vi "CalcDivergence.vi"(6 "AOI":cluster{"AOI h, px":dbl, "AOI w, px":dbl}, 7 "Rotate, deg":dbl=1.6 format="%#_13g", 8 "Focus, mm":dbl=192.0, 9 "Pixel size, um":dbl=6.45, 10 "Threshold, %":dbl=85.0 format="%#_13g", 11 "path to file":path=path "E:/New folder (3)/Laser(3dots)_FarField_after_Passive(WO_SAC).png") -> (2 "Slow Axis":T1, 3 "Fast Axis":T1)   [LabVIEW 2017]
panel:
  out "Picture":picture
  in  "Zoom Factor":sgl=0.4
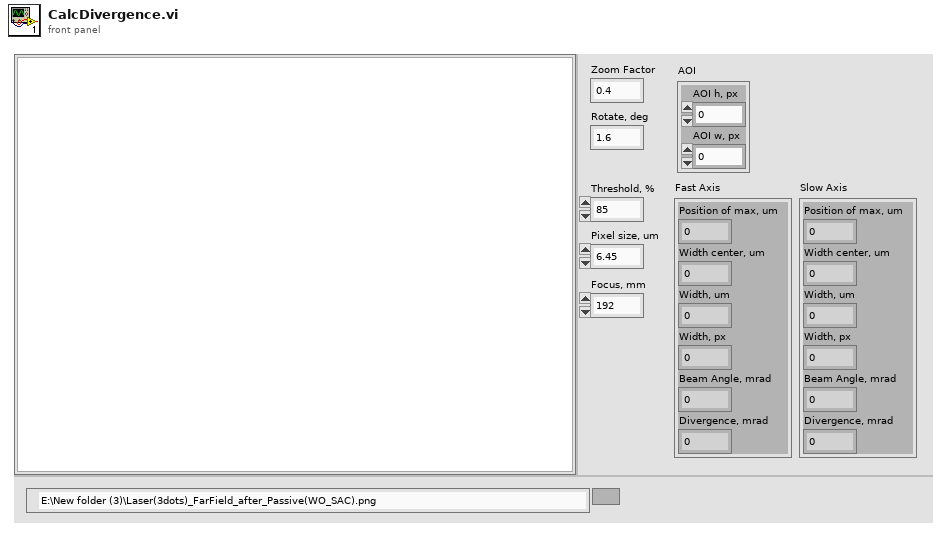
[diagram p1: front panel]
types:
  T1 = cluster{"Position of max, um":dbl, "Width center, um":dbl, "Width, um":dbl, "Width, px":i32, "Beam Angle, mrad":dbl, "Divergence, mrad":dbl}
  T2 = typedef "imagedata.ctl" = cluster{"image type":i32, "image depth":i32, "image":u8[], "mask":u8[], "colors":u32[], "Rectangle":cluster{"left":i16, "top":i16, "right":i16, "bottom":i16}}
  T3 = cluster{"Centroid of max, um":dbl, "Centroid of width, um":dbl, "Width, um":dbl, "Width, px":i32, "Beam Angle, mrad":dbl, "Divergence, mrad":dbl}
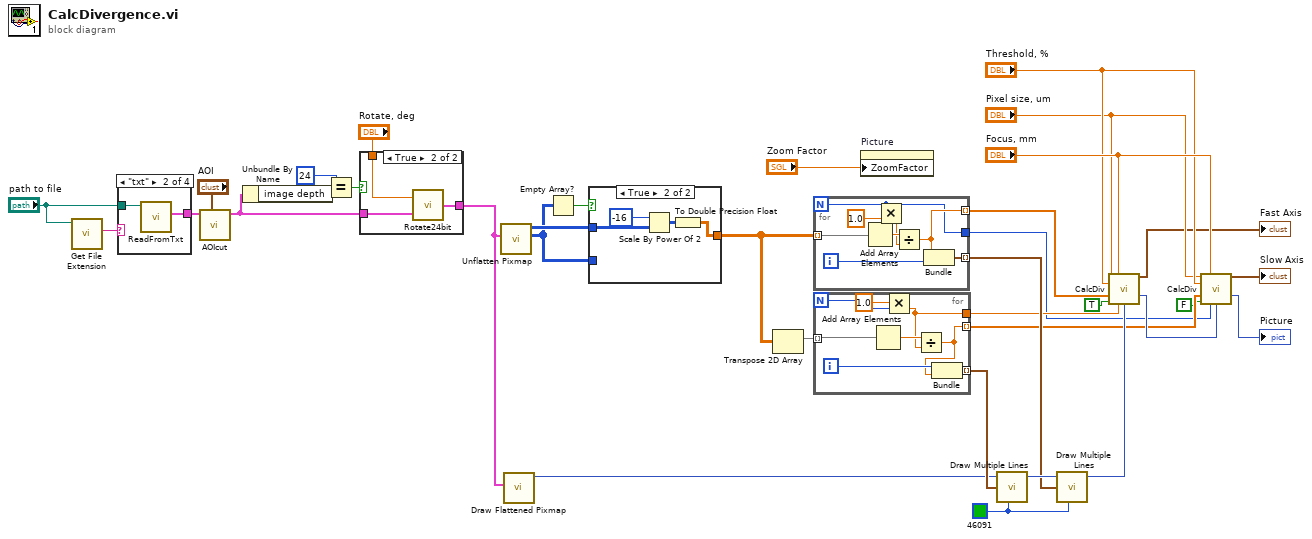
[diagram p0: block diagram]
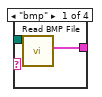
[diagram p2: hidden frame]
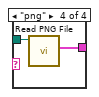
[diagram p4: hidden frame]
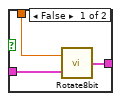
[diagram p5: hidden frame]
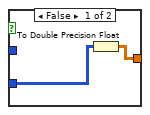
[diagram p6: hidden frame]
diagram:
  w26 = u32 46091 ("color(black)")
  n1 = call <vilib>:"Get File Extension.vi"("file"="path to file") -> ("lowercase file extension"=w7:string)  [unwired: 6 in, 4 out]
  n2 = case shown="\"txt\"" w7 {
    tunnel: [w36 w38 _ w41] -> w6
    tunnel: "path to file" -> [w37 w39 _ w40]
    frame "bmp" {
      n3 = call <vilib>:"Read BMP File.vi"("path to BMP file"=w37) -> ("image data"=w36:T2)  [unwired: 8 in, 2 out]
    }
    frame "txt" {
      n4 = call "ReadFromTxt.vi"("path to PNG file"=w39) -> ("image data"=w38:T2)  [unwired: 10 in]
    }
    frame Default {
    }
    frame "png" {
      n5 = call <vilib>:"Read PNG File.vi"("path to PNG file"=w40) -> ("image data"=w41:T2)  [unwired: 8 in, 2 out]
    }
  }
  n6 = call "AOIcut.vi"("AOI"="AOI", "image data in"=w6) -> ("image data out"=w3:T2)  [unwired: 9 in]
  n7 = Unbundle By Name(w3) -> ("image depth"=w10:i32)
  n8 = Equal?(x=24, y=w10) -> (x = y?=w8:bool)
  n9 = case shown="True" w8 {
    tunnel: "Rotate, deg" -> [w44 w47]
    tunnel: [w42 w46] -> w30
    tunnel: w3 -> [w43 w45]
    frame False {
      n10 = call "Rotate8bit.vi"("image data"=w43, "theta (deg)"=w44) -> ("image data 2"=w42:T2)
    }
    frame True {
      n11 = call "Rotate24bit.vi"("image data"=w45, "theta (deg)"=w47) -> ("image data 2"=w46:T2)
    }
  }
  n12 = call <vilib>:"Unflatten Pixmap.vi"("image data"=w30) -> ("8-bit pixmap"=w12:u8[][], "24-bit pixmap"=w14:u32[][])  [unwired: 4 in, 5 out]
  n13 = call <vilib>:"Draw Flattened Pixmap.vi"("image data"=w30) -> ("new picture"=w29:picture)  [unwired: 8 in]
  n14 = Empty Array?(array=w12) -> (empty?=w11:bool)
  n15 = case shown="True" w11 {
    tunnel: w14 -> [_ w53]
    tunnel: [w49 w50] -> w13
    tunnel: w12 -> [w48 _]
    frame False {
      n16 = To Double Precision Float(number=w48) -> (double precision float=w49:dbl[][])
    }
    frame True {
      n17 = Scale By Power Of 2(n=i16 -16, x=w53) -> (x*2^n=w51:u32[][])
      n18 = To Double Precision Float(number=w51) -> (double precision float=w50:dbl[][])
    }
  }
  n19 = Transpose 2D Array(2D array=w13) -> (transposed array=w33:dbl[][])
  n20 = for {
    N -> [w57]
    tunnel: w13 -> [w56] mode=indexing
    tunnel: [w60] -> w28 mode=indexing
    tunnel: [w58] -> w25 mode=indexing
    tunnel: [w57] -> w19
    i -> [w61]
    n21 = Add Array Elements(numeric array=w56) -> (sum=w59:dbl)
    n22 = Multiply(x=w57, y=1.0) -> (x*y=w55:dbl)
    n23 = Divide(x=w59, y=w55) -> (x/y=w58:dbl)
    n24 = Bundle(w58, w61) -> (w60:cluster{dbl, i32})  [unwired: 1 in]
  }
  n25 = for {
    N -> [w66]
    tunnel: w33 -> [w64] mode=indexing
    tunnel: [w68] -> w32 mode=indexing
    tunnel: [w63] -> w24
    tunnel: [w65] -> w20 mode=indexing
    i -> [w69]
    n26 = Add Array Elements(numeric array=w64) -> (sum=w67:dbl)
    n27 = Multiply(x=1.0, y=w66) -> (x*y=w63:dbl)
    n28 = Divide(x=w67, y=w63) -> (x/y=w65:dbl)
    n29 = Bundle(w69, w65) -> (w68:cluster{i32, dbl})  [unwired: 1 in]
  }
  n30 = property on="Picture" class="Pict"("ZoomFactor"="Zoom Factor") -> ()  [unwired: 2 in, 2 out]
  n31 = call <vilib>:"Draw Multiple Lines.vi"("picture"=w29, "line endpoints"=w32, "color(black)"=w26) -> ("new picture"=w31:picture)  [unwired: 6 in]
  n32 = call <vilib>:"Draw Multiple Lines.vi"("picture"=w31, "line endpoints"=w28, "color(black)"=w26) -> ("new picture"=w27:picture)  [unwired: 6 in]
  n33 = call "CalcDiv.vi"("Pixel size, um"="Pixel size, um", "Focus, mm"="Focus, mm", "Threshold, %"="Threshold, %", "Array"=w25, "SAC/FAC"=TRUE, "Numeric in"=w24, "new picture in"=w27) -> ("Beam Params"=→"Fast Axis":T3, "new picture out"=w23:picture)  [unwired: 7 in]
  n34 = call "CalcDiv.vi"("Pixel size, um"="Pixel size, um", "Focus, mm"="Focus, mm", "Threshold, %"="Threshold, %", "Array"=w20, "SAC/FAC"=FALSE, "Numeric in"=w19, "new picture in"=w23) -> ("Beam Params"=→"Slow Axis":T3, "new picture out"=→"Picture":picture)  [unwired: 7 in]
